vi "查询数据.vi"(5 "condition":string, 6 "Distinct":bool, 7 "columns":string[](array[string]), 8 "error in (no error)":errorcluster, 10 "database":string="database1.mdb", 11 "table":string) -> (0 "error out":errorcluster, 3 "data":variant[][](array[variant]))   [LabVIEW 2016, in "数据查询.lvlib"]
uses:
  <vilib>/addons/database/Connection.llb/DB Tools Open Connec (String).vi
  <vilib>/addons/database/NI_Database_API.lvlib
  database/Access/Access Lib.lvlib
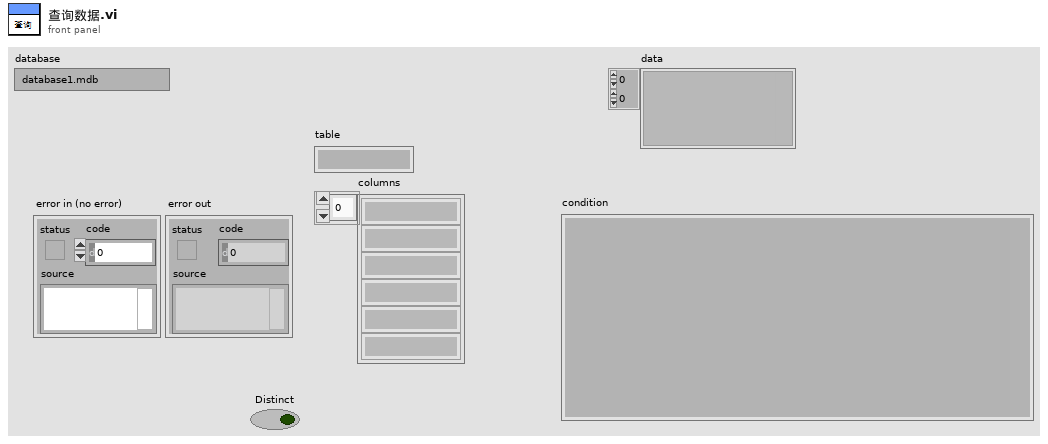
[diagram p1: front panel]
types:
  T1 = typedef "NI_Database_API.lvlib/Conn ObjectReference.ctl" = refnum<k1>
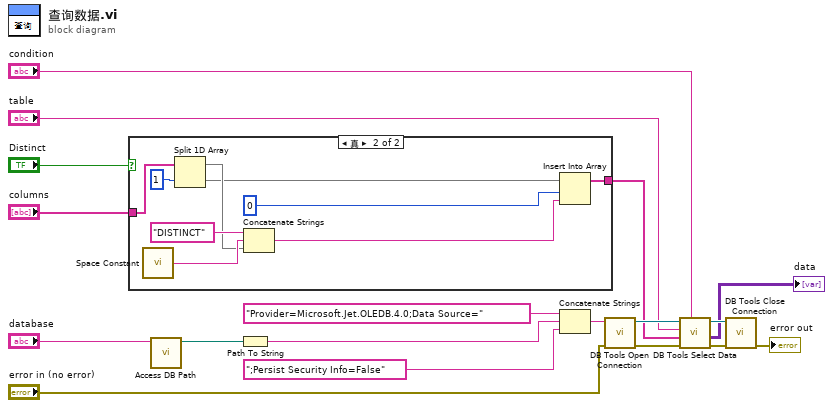
[diagram p0: block diagram]
diagram:
  n1 = case shown="真" "Distinct" {
    tunnel: "columns" -> [w19 w28]
    tunnel: [w19 w22] -> w3
    frame False {
    }
    frame True {
      n2 = call <vilib>:"Space Constant.vi"() -> ("String"=w25:string)
      n3 = Split 1D Array(array=w28, index=1 ("索引")) -> (first subarray=w21:string[], second subarray=w20:string[])
      n4 = Concatenate Strings("DISTINCT" ("字符串"), w25, w21) -> (w27:string)
      n5 = Insert Into Array(array=w20, index=0 ("索引"), new element=w27) -> (w22:string[])
    }
  }
  n6 = call "Access DB Path.vi"("database"="database") -> ("appended path"=w1:path)  [unwired: 10 in]
  n7 = Path To String(path=w1) -> (string=w10:string)
  n8 = Concatenate Strings("Provider=Microsoft.Jet.OLEDB.4.0;Data Source=" ("condition"), w10, ";Persist Security Info=False" ("condition")) -> (w8:string)
  n9 = call-poly <vilib>:"DB Tools Open Connection.vi"("error in (no error)"="error in (no error)", "connection information"=w8) -> ("error out"=w16:errorcluster, "connection reference"=w18:T1)  [unwired: 6 in]
  n10 = call <vilib>:"DB Tools Select Data.vi"("condition"="condition", "error in (no error)"=w16, "columns"=w3, "table"="table", "connection reference"=w18) -> ("error out"=w15:errorcluster, "data"=→"data":variant[][], "connection reference out"=w17:T1)  [unwired: 1 in]
  n11 = call <vilib>:"DB Tools Close Connection.vi"("error in (no error)"=w15, "connection reference"=w17) -> ("error out"=→"error out":errorcluster)  [unwired: 5 in]
